vi "Add Child Items to Tree.vi"(8 "error in (no error)":errorcluster, 10 "Standard VI Type in":refnum<class "Standard VI Type.lvclass">, 11 "Tree Ref in":refnum<vi>) -> (0 "error out":errorcluster, 2 "Standard VI Type out":refnum<class "Standard VI Type.lvclass">, 3 "Tree Ref out":refnum<vi>)   [LabVIEW 2020, in "Peek Window.lvlib" / "Standard VI Type.lvclass"]
uses:
  Standard VI Type.lvclass
  Standard VI Type.lvclass/Standard VI Type.ctl
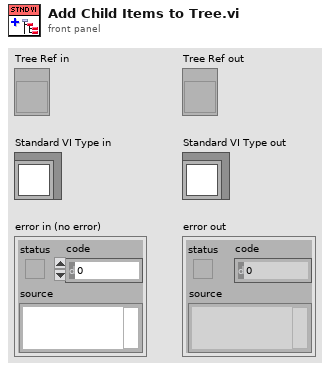
[diagram p1: front panel]
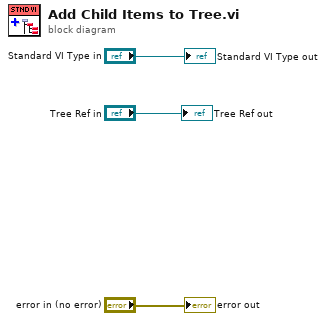
[diagram p0: block diagram]
diagram:
  "error out" <- "error in (no error)"
  "Tree Ref out" <- "Tree Ref in"
  "Standard VI Type out" <- "Standard VI Type in"
